vi "EXCOM-25.vi"(0 "VISA resource name":refnum<visa-resource-name>, 2 "Bool Refnum":refnum<vi>) -> (5 "OK Done":bool, 6 "HA":dbl format="%<%H:%M:%S%0u>t", 7 "Q String":string, 8 "RA":dbl format="%<%H:%M:%S%0u>t", 9 "Rotateur":dbl format="%.2f", 10 "DEC":dbl format="%<%H:%M:%S%0u>t", 11 "Dome":dbl format="%.2f", 12 "Epoque":dbl format="%.2f", 13 "Focus":dbl format="%.2f", 14 "VISA resource name dup":refnum<visa-resource-name>, 15 "Masse d'air":dbl format="%.2f", 16 "Temps Sidéral":dbl format="%<%H:%M:%S%0u>t", 17 "Temps Universel":dbl format="%<%H:%M:%S%0u>t", 18 "Année":dbl format="%.2f", 19 "Error OUT":errorcluster)   [LabVIEW 2011]
panel:
  in  "Error IN":errorcluster
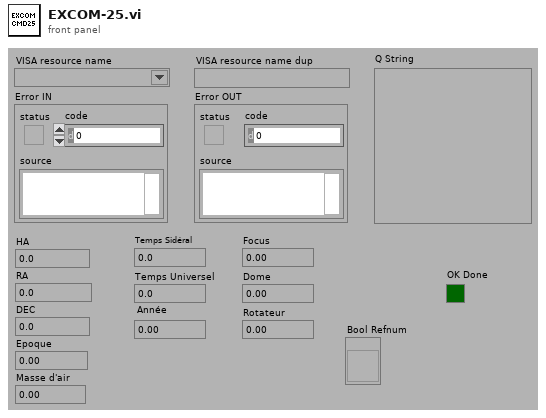
[diagram p1: front panel]
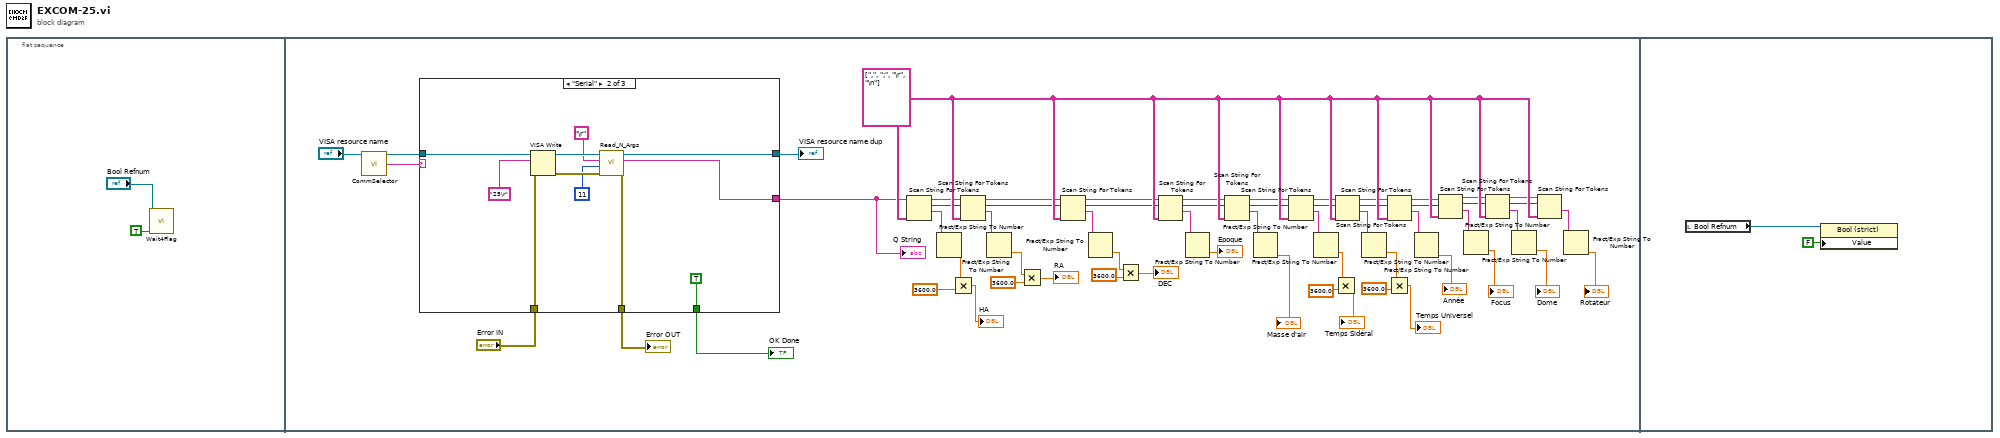
[diagram p0: block diagram]
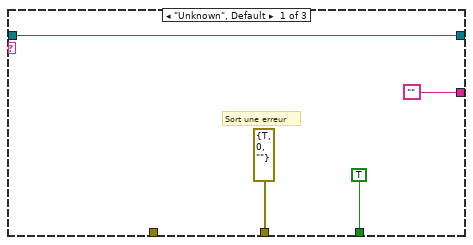
[diagram p2: hidden frame]
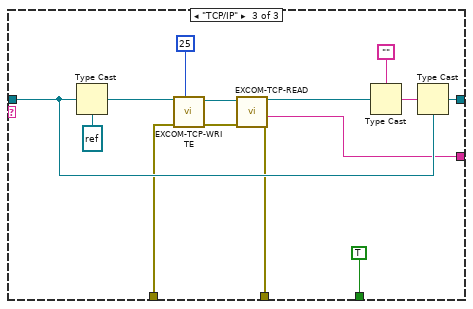
[diagram p3: hidden frame]
diagram:
  n1 = flat-sequence {
    frame #0 {
      n2 = call "Wait4Flag.vi"("Raise Flag ?"=TRUE, "Ctl Refnum IN"="Bool Refnum") -> ()  [unwired: 8 in, 2 out]
    }
    frame #1 {
      w55 = string[] [",", ";", "\r", "\n"] ("delimiters (\\s,\\t,\\r,\\n)")
      n3 = call "CommSelector.vi"("VISA resource name"="VISA resource name") -> ("VISA resource name"=w58:refnum<visa-resource-name>, "CommType"=w57:string)  [unwired: 13 in]
      n4 = case shown="\"Serial\"" w57 {
        tunnel: w58 -> [w65 w70 w87]
        tunnel: [TRUE ("OK Done") TRUE ("OK Done") TRUE ("OK Done")] -> w63
        tunnel: [errorcluster {"status"=TRUE, "code"=0, "source"=""} ("error out") w77 w81] -> w62
        tunnel: [w65 w71 w86] -> w61
        tunnel: "Error IN" -> [_ w69 w82]
        tunnel: ["" w68 w79] -> w3
        frame "Unknown", Default {
          # "Sort une erreur"
        }
        frame "Serial" {
          n5 = VISA Write(VISA resource name=w70, write buffer="25\r" ("String to Send"), error in (no error)=w69) -> (VISA resource name out=w75:refnum<visa-resource-name>, error out=w76:errorcluster)  [unwired: 1 out]
          n6 = call "Read_N_Args.vi"("Error IN"=w76, "Nb_Args"=11, "Arg_Char"="\r", "VRN IN"=w75) -> ("Error OUT"=w77:errorcluster, "Answer"=w68:string, "VRN OUT"=w71:refnum<visa-resource-name>)  [unwired: 4 in, 1 out]
        }
        frame "TCP/IP" {
          n7 = Type Cast(type=refnum<k5> refnum ("CID Out"), x=w87) -> (*(type *) &x=w88:refnum<k5>)
          n8 = call "EXCOM-TCP-WRITE.vi"("Commande #"=25, "Error IN"=w82, "connection ID"=w88) -> ("Error OUT"=w92:errorcluster, "connection ID out"=w91:refnum<k5>)  [unwired: 4 in, 2 out]
          n9 = call "EXCOM-TCP-READ.vi"("Error In"=w92, "connection ID"=w91) -> ("Error Out"=w81:errorcluster, "Response"=w79:string, "CID Out"=w85:refnum<k5>)  [unwired: 5 in]
          n10 = Type Cast(type="", x=w85) -> (*(type *) &x=w83:string)
          n11 = Type Cast(type=w87, x=w83) -> (*(type *) &x=w86:refnum<visa-resource-name>)
        }
      }
      "VISA resource name dup" <- w61
      "OK Done" <- w63
      "Error OUT" <- w62
      "Q String" <- w3
      n12 = Scan String For Tokens(6:w55, 9:w3) -> (1:w12:string, 2:w11:i32, 3:w10:string)  [unwired: 4 in, 1 out]
      n13 = Fract/Exp String To Number(string=w12) -> (number=w13:dbl)  [unwired: 3 in, 1 out]
      n14 = Multiply(x=w13, y=3600.0) -> (x*y=→"HA":dbl)
      n15 = Scan String For Tokens(6:w55, 8:w11, 9:w10) -> (1:w54:string, 2:w8:i32, 3:w9:string)  [unwired: 3 in, 1 out]
      n16 = Fract/Exp String To Number(string=w54) -> (number=w21:dbl)  [unwired: 3 in, 1 out]
      n17 = Multiply(x=w21, y=3600.0) -> (x*y=→"RA":dbl)
      n18 = Scan String For Tokens(6:w55, 8:w8, 9:w9) -> (1:w18:string, 2:w6:i32, 3:w7:string)  [unwired: 3 in, 1 out]
      n19 = Fract/Exp String To Number(string=w18) -> (number=w23:dbl)  [unwired: 3 in, 1 out]
      n20 = Multiply(x=w23, y=3600.0) -> (x*y=→"DEC":dbl)
      n21 = Scan String For Tokens(6:w55, 8:w6, 9:w7) -> (1:w19:string, 2:w4:i32, 3:w5:string)  [unwired: 3 in, 1 out]
      n22 = Fract/Exp String To Number(string=w19) -> (number=→"Epoque":dbl)  [unwired: 3 in, 1 out]
      n23 = Scan String For Tokens(6:w55, 8:w4, 9:w5) -> (1:w20:string, 2:w52:i32, 3:w33:string)  [unwired: 3 in, 1 out]
      n24 = Fract/Exp String To Number(string=w20) -> (number=→"Masse d'air":dbl)  [unwired: 3 in, 1 out]
      n25 = Scan String For Tokens(6:w55, 8:w52, 9:w33) -> (1:w28:string, 2:w30:i32, 3:w29:string)  [unwired: 3 in, 1 out]
      n26 = Fract/Exp String To Number(string=w28) -> (number=w25:dbl)  [unwired: 3 in, 1 out]
      n27 = Multiply(x=w25, y=3600.0) -> (x*y=→"Temps Sidéral":dbl)
      n28 = Scan String For Tokens(6:w55, 8:w30, 9:w29) -> (1:w27:string, 2:w32:i32, 3:w31:string)  [unwired: 3 in, 1 out]
      n29 = Fract/Exp String To Number(string=w27) -> (number=w24:dbl)  [unwired: 3 in, 1 out]
      n30 = Scan String For Tokens(6:w55, 8:w32, 9:w31) -> (1:w26:string, 2:w53:i32, 3:w43:string)  [unwired: 3 in, 1 out]
      n31 = Multiply(x=w24, y=3600.0) -> (x*y=→"Temps Universel":dbl)
      n32 = Fract/Exp String To Number(string=w26) -> (number=→"Année":dbl)  [unwired: 3 in, 1 out]
      n33 = Scan String For Tokens(6:w55, 8:w53, 9:w43) -> (1:w40:string, 2:w38:i32, 3:w39:string)  [unwired: 3 in, 1 out]
      n34 = Fract/Exp String To Number(string=w40) -> (number=→"Focus":dbl)  [unwired: 3 in, 1 out]
      n35 = Scan String For Tokens(6:w55, 8:w38, 9:w39) -> (1:w41:string, 2:w36:i32, 3:w37:string)  [unwired: 3 in, 1 out]
      n36 = Fract/Exp String To Number(string=w41) -> (number=→"Dome":dbl)  [unwired: 3 in, 1 out]
      n37 = Scan String For Tokens(6:w55, 8:w36, 9:w37) -> (1:w42:string)  [unwired: 3 in, 3 out]
      n38 = Fract/Exp String To Number(string=w42) -> (number=→"Rotateur":dbl)  [unwired: 3 in, 1 out]
    }
    frame #2 {
      n39 = local read "Bool Refnum"() -> (w94:refnum<vi>)
      n40 = property on="Property Node" class="Bool (strict)"(reference=w94, "Value"=FALSE) -> ()  [unwired: 1 in, 2 out]
    }
  }
